vi "Get Transfer Configuration.vi"(8 "error in":errorcluster, 11 "Component Configuration in":refnum<class "RDMA Configurations.lvclass">=refnum) -> (0 "error out":errorcluster, 1 "Tx Transfer Configuration":refnum<class "Configuration.lvclass">, 2 "Rx Transfer Configuration":refnum<class "Configuration.lvclass">, 3 "Component Configuration out":refnum<class "RDMA Configurations.lvclass">)   [LabVIEW 2020, in "RDMA.lvlib" / "RDMA Configurations.lvclass"]
uses:
  RDMA Configurations.lvclass
  Rx Transfer/RDMA Transfer Rx Configuration.lvclass
  Tx Transfer/RDMA Transfer Tx Configuration.lvclass
  DSF Core.lvlibp/Classes/Configuration/Configuration.lvclass
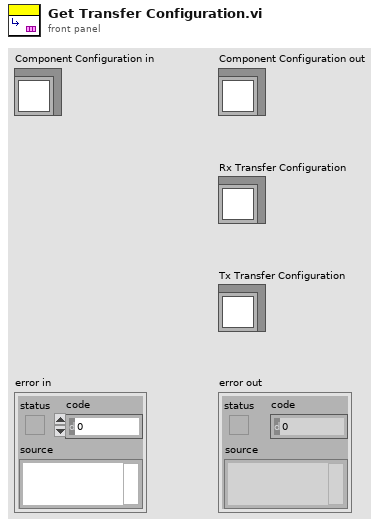
[diagram p1: front panel]
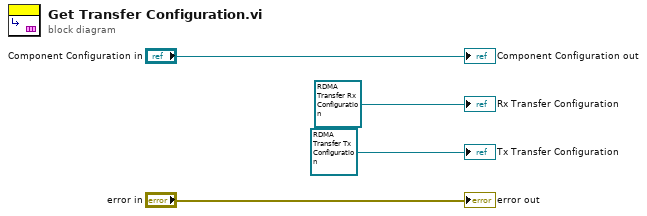
[diagram p0: block diagram]
diagram:
  "error out" <- "error in"
  "Component Configuration out" <- "Component Configuration in"
  "Rx Transfer Configuration" <- refnum<class "RDMA Transfer Rx Configuration.lvclass"> refnum ("RDMA.lvlib:RDMA Transfer Rx Configuration.lvclass")
  "Tx Transfer Configuration" <- refnum<class "RDMA Transfer Tx Configuration.lvclass"> refnum ("RDMA.lvlib:RDMA Transfer Tx Configuration.lvclass")
